vi "Event--Shortcut Menu Activation.vi"(8 "error in":errorcluster, 9 "Coords":T1, 10 "MenuRef":refnum<k9>, 11 "Selector in":refnum<class "Selector.lvclass">) -> (0 "error out":errorcluster, 3 "Selector out":refnum<class "Selector.lvclass">)   [LabVIEW 2019, in "Selector.lvclass"]
uses:
  Selector.lvclass
  <vilib>/Utility/miscctls.llb/LVPoint32TypeDef.ctl
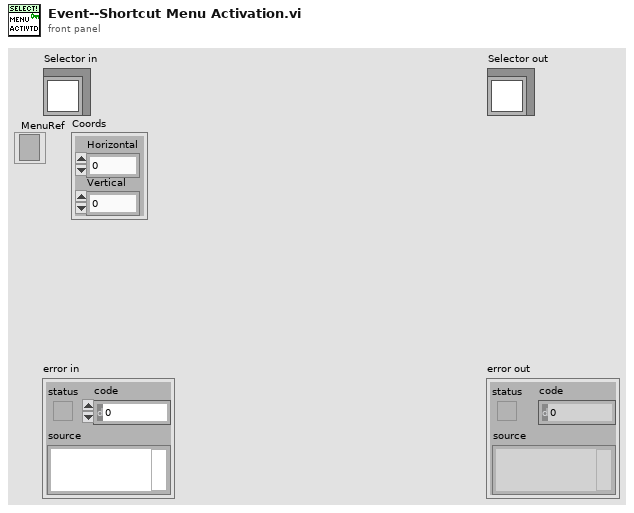
[diagram p1: front panel]
types:
  T1 = typedef "LVPoint32TypeDef.ctl" = cluster{"Horizontal":i32, "Vertical":i32}
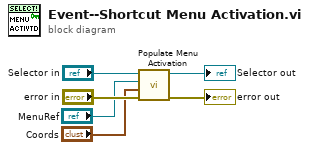
[diagram p0: block diagram]
diagram:
  n1 = call-dynamic "Populate Menu Activation.vi"("error in (no error)"="error in", "Point32"="Coords", "MenuRef"="MenuRef", "Selector in"="Selector in") -> ("error out"=→"error out":errorcluster, "Selector out"=→"Selector out":refnum<class "Selector.lvclass">)  [unwired: 6 in]
